vi "Get.vi"(8 "error in (no error)":errorcluster, 10 "Key":variant, 11 "Store in":refnum<class "Store.lvclass">) -> (0 "error out":errorcluster, 1 "Success?":bool, 2 "Value":variant, 3 "Store out":refnum<class "Store.lvclass">)   [LabVIEW 2018, in "Application.lvlib" / "Store.lvclass"]
uses:
  Store.lvclass
  Store.lvclass/Store.ctl
  Controls/Packet.ctl
  Dictionary Class/Dictionary.lvclass/Dictionary.ctl
  Dictionary Class/VIs/Get Data DVR.vi
  Dictionary Class/Dictionary.lvclass
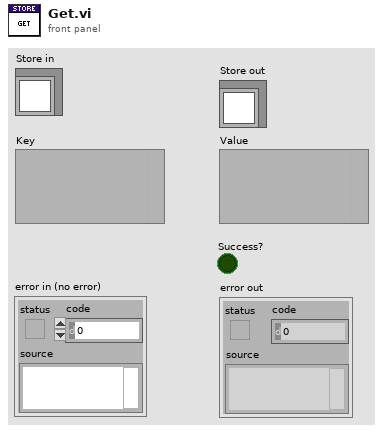
[diagram p1: front panel]
types:
  T1 = typedef "Application.lvlib/Store.lvclass/Packet.ctl" = cluster{"Type Descriptor":i16[], "Value":variant}
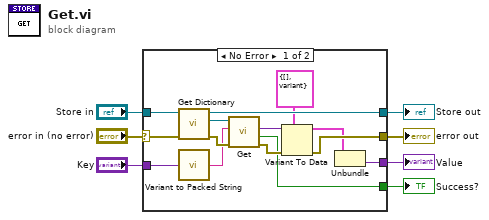
[diagram p0: block diagram]
diagram:
  n1 = case shown="No Error" "error in (no error)" {
    selector: "error in (no error)" -> [w20 w23]
    tunnel: [w9 w23] -> w6
    tunnel: [w18 w22] -> w4
    tunnel: "Store in" -> [w21 w22]
    tunnel: "Key" -> [w19 _]
    tunnel: [w17 _] -> w2
    tunnel: [w11 _] -> w1
    frame No Error {
      n2 = call "Get Dictionary.vi"("error in (no error)"=w20, "Store in"=w21) -> ("error out"=w15:errorcluster, "Dictionary.lvclass"=w16:refnum<class "Dictionary.lvclass">, "Store out"=w18:refnum<class "Store.lvclass">)  [unwired: 7 in]
      n3 = call "Variant to Packed String.vi"("Variant"=w19) -> ("Packed String"=w14:string)  [unwired: 3 in, 1 out]
      n4 = call "Get.vi"("error in (no error)"=w15, "Key"=w14, "Dictionary in"=w16) -> ("error out"=w13:errorcluster, "Success?"=w11:bool, "Value"=w12:variant)  [unwired: 5 in, 1 out]
      n5 = Variant To Data(error in=w13, type=T1 {"Type Descriptor"=[], "Value"=variant} ("Packet"), Variant=w12) -> (data=w8:T1, error out=w9:errorcluster)
      n6 = Unbundle(w8) -> ("Value"=w17:variant)  [unwired: 1 out]
    }
    frame Error {
    }
  }
  "error out" <- w6
  "Store out" <- w4
  "Value" <- w2
  "Success?" <- w1
